vi "Server Client Loop.vi"(5 "TCPMessageAPI":refnum<class "TCPMessageAPI.lvclass">, 6 "Client Action Q":refnum<queue>, 7 "Fwd Queue":refnum<queue>, 8 "TCP Client":refnum<k5>, 9 "Remote Port":u16, 10 "Remote Address":string, 11 "Conn Handlers":refnum<queue>) -> ()   [LabVIEW 2020, in "Vecto.lvlib" / "TCPMessaging.lvclass"]
uses:
  TCPMessaging.lvclass
  TX Payload.ctl
  Client Action Data.ctl
  Client Action.ctl
  Client Info.ctl
  proto/TcpClientHello/Data.ctl
  TCPMessageService/TCPMessageAPI.lvclass
  TCPConnectionHandler/TCPConnectionHandler.lvclass
  Server Client State.ctl
  Connection State.ctl
  Vecto.lvlib
  proto/TcpClientHello/TcpClientHello.lvlib
panel:
  out "Client Hello":T1
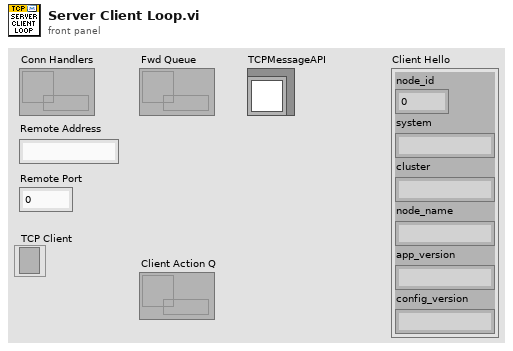
[diagram p1: front panel]
types:
  T1 = typedef "TcpClientHello.lvlib/Data.ctl" = cluster{"node_id":u32, "system":string, "cluster":string, "node_name":string, "app_version":string, "config_version":string}
  T2 = typedef "Vecto.lvlib/TCPMessaging.lvclass/Server Client State.ctl" = enum16{"Handshake", "Message", "Close"}
  T3 = enum16{"big-endian, network order", "native, host order", "little-endian"}
  T4 = typedef "Vecto.lvlib/TCPMessaging.lvclass/Client Action.ctl" = enum16{"Connect", "Ready", "Disconnect"}
  T5 = typedef "Vecto.lvlib/TCPMessaging.lvclass/Client Action Data.ctl" = cluster{"Client Action":T4, "Client Info":T6, "TCP":refnum<k5>, "TX Q":refnum<queue>}
  T6 = typedef "Vecto.lvlib/Client Info.ctl" = cluster{"TcpClientHello":T1, "Remote Address":string, "Remote Port":u16}
  T7 = typedef "Vecto.lvlib/Connection State.ctl" = enum16{"Connected", "Disconnected"}
  T8 = typedef "Vecto.lvlib/TX Payload.ctl" = cluster{"Target ID":u32, "Payload":string}
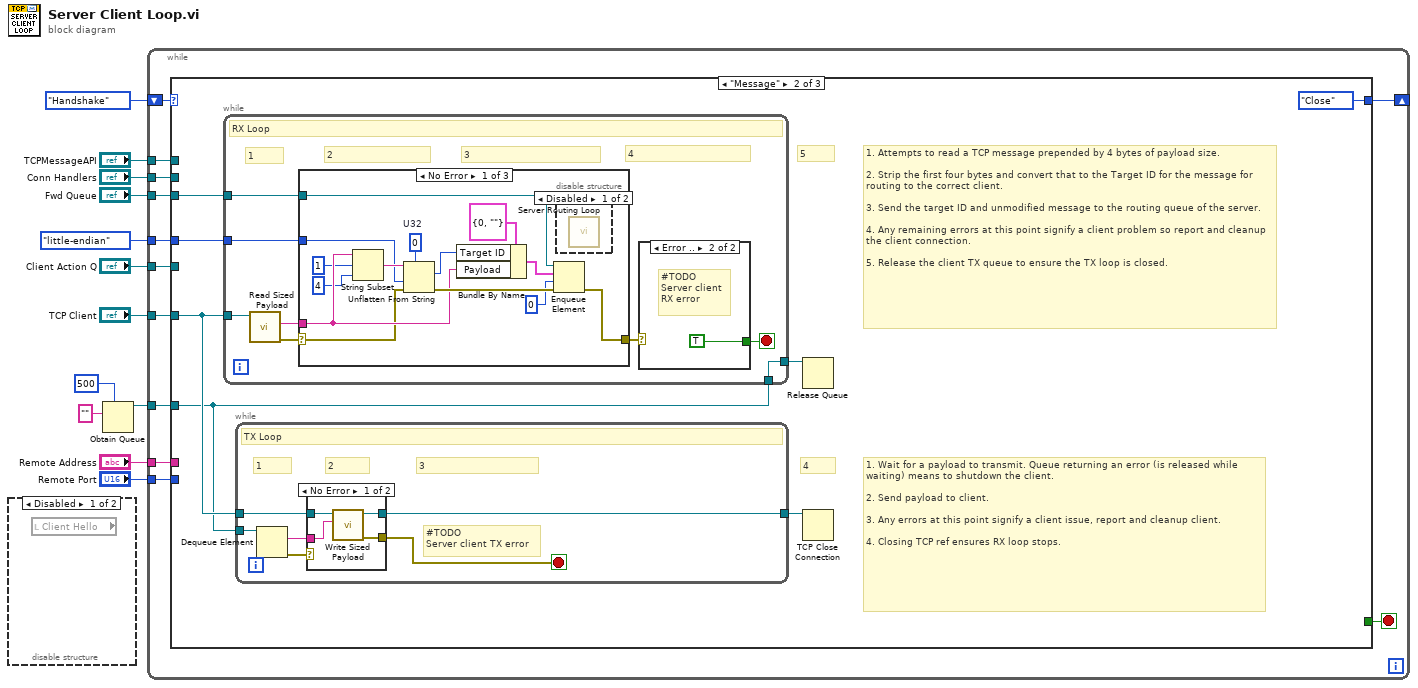
[diagram p0: block diagram]
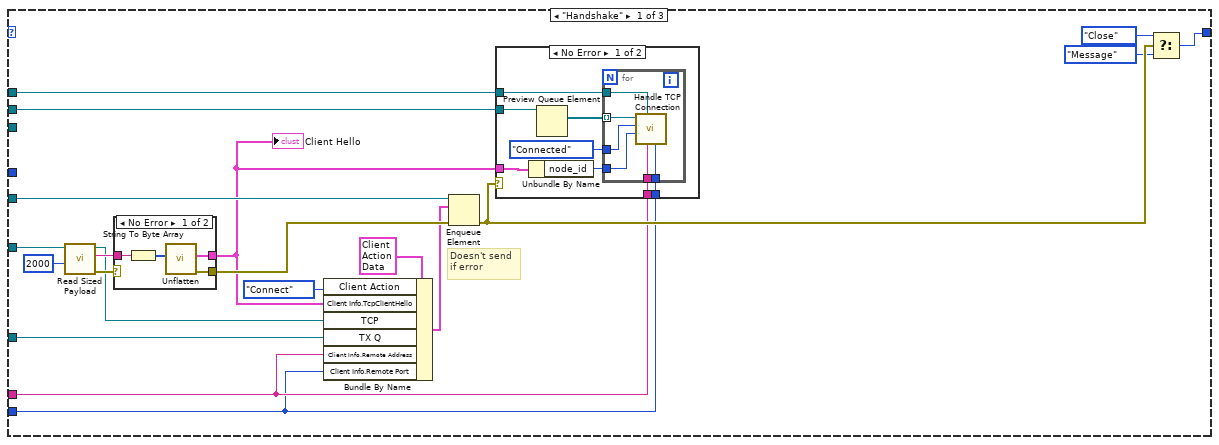
[diagram p3: hidden frame]
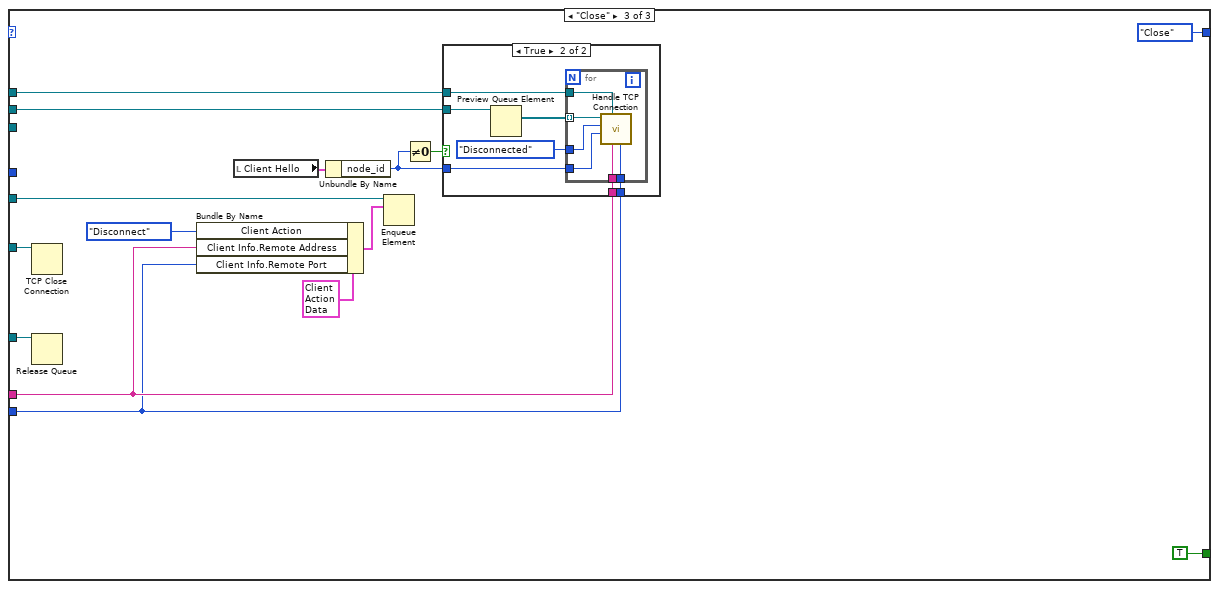
[diagram p11: hidden frame]
diagram:
  n1 = disable-structure shown="Disabled" {
    frame Disabled {
      n2 = local read "Client Hello"() -> ()  [unwired: 1 out]
    }
    frame Enabled {
    }
  }
  n3 = Obtain Queue(max queue size (-1, unlimited)=500, element data type="") -> (queue out=w4:refnum<queue>)  [unwired: 3 in, 2 out]
  n4 = while {
    tunnel: "Fwd Queue" -> [w24]
    tunnel: "TCP Client" -> [w23]
    tunnel: T3."little-endian" ("byte order (0:big-endian, network order)") -> [w22]
    shift-right: [w19] -> _
    shift-left: Server_Client_State."Handshake" ("Server Client State") -> [w20]
    tunnel: "Remote Address" -> [w18]
    tunnel: "Remote Port" -> [w17]
    tunnel: w4 -> [w16]
    tunnel: "Client Action Q" -> [w15]
    tunnel: "Conn Handlers" -> [w14]
    tunnel: "TCPMessageAPI" -> [w13]
    stop <- w21 stop-if-true
    n5 = case shown="\"Message\"" w20 {
      tunnel: w24 -> [_ w70 _]
      tunnel: w23 -> [w39 w69 w118]
      tunnel: w22 -> [_ w68 _]
      tunnel: [_ _ TRUE] -> w21
      tunnel: [w40 Server_Client_State."Close" ("Server Client State") Server_Client_State."Close" ("Server Client State")] -> w19
      tunnel: w18 -> [w26 _ w108]
      tunnel: w17 -> [w25 _ w107]
      tunnel: w16 -> [w30 w64 w119]
      tunnel: w15 -> [w35 _ w116]
      tunnel: w14 -> [w29 _ w113]
      tunnel: w13 -> [w28 _ w112]
      frame "Handshake" {
        # "Doesn't send if error"
        n6 = call "Read Sized Payload.vi"("timeout ms (100)"=2000, "TCP in"=w39) -> ("error out"=w37:errorcluster, "Payload"=w36:string, "TCP"=w32:refnum<k5>)  [unwired: 7 in]
        n7 = case shown="No Error" w37 {
          selector: w37 -> [_ w63]
          tunnel: w36 -> [w62 _]
          tunnel: [w60 _] -> w27
          tunnel: [w59 w63] -> w43
          frame No Error {
            n8 = String To Byte Array(string=w62) -> (unsigned byte array=w61:u8[])
            n9 = call "Unflatten.vi"("Buffer"=w61) -> ("error out"=w59:errorcluster, "Data"=w60:T1)  [unwired: 9 in]
          }
          frame Error {
          }
        }
        "Client Hello" <- w27
        n10 = Bundle By Name(cluster=T5 {"Client Action"=enum."Disconnect", "Client Info"={"TcpClientHello"={"node_id"=0, "system"="", "cluster"="", "node_name"="", "app_version"="", "config_version"=""}, "Remote Address"="", "Remote Port"=0}, "TCP"=refnum, "TX Q"=refnum} ("element"), "Client Action"=Client_Action."Connect", "Client Info.TcpClientHello"=w27, "TCP"=w32, "TX Q"=w30, "Client Info.Remote Address"=w26, "Client Info.Remote Port"=w25) -> (w31:T5)
        n11 = Enqueue Element(queue=w35, element=w31, error in (no error)=w43) -> (error out=w44:errorcluster)  [unwired: 1 in, 2 out]
        n12 = case shown="No Error" w44 {
          tunnel: w29 -> [w48 _]
          tunnel: w27 -> [w52 _]
          tunnel: w28 -> [w51 _]
          tunnel: w26 -> [w46 _]
          tunnel: w25 -> [w45 _]
          frame No Error {
            n13 = Unbundle By Name(w52) -> ("node_id"=w50:u32)
            n14 = Preview Queue Element(queue=w48) -> (element=w47:refnum<class "TCPConnectionHandler.lvclass">[])  [unwired: 2 in, 3 out]
            n15 = for {
              tunnel: w47 -> [w58] mode=indexing
              tunnel: w51 -> [w57]
              tunnel: w50 -> [w55]
              tunnel: Connection_State."Connected" ("Connection State") -> [w56]
              tunnel: w46 -> [w54]
              tunnel: w45 -> [w53]
              n16 = call-dynamic "Handle TCP Connection.vi"("Remote Port"=w53, "Remote Host"=w54, "TCPMessageAPI"=w57, "Node ID"=w55, "Connection State"=w56, "TCPConnectionHandler in"=w58) -> ()  [unwired: 4 in, 2 out]
            }
          }
          frame Error {
          }
        }
        n17 = Select(t=Server_Client_State."Close", s=w44, f=Server_Client_State."Message" ("Server Client State")) -> (s? t:f=w40:T2)
      }
      frame "Message" {
        # "4"
        # "5"
        # "1. Wait for a payload to transmit. Queue returning an error (is released while waiting) means to shutdown the client.\n\n2. Send payload to client.\n\n3. Any errors at this point signify a client issue, report and cleanup client.\n\n4. Closing TCP ref ensures RX loop stops."
        # "1. Attempts to read a TCP message prepended by 4 bytes of payload size.\n\n2. Strip the first four bytes and convert that to the Target ID for the message for routing to the correct client.\n\n3. Send the target ID and unmodified message to the routing queue of the server.\n\n4. Any remaining errors at this point signify a client problem so report and cleanup the client connection.\n\n5. Release the client TX queue to ensure the TX loop is closed."
        n18 = while {
          tunnel: w70 -> [w78]
          tunnel: w69 -> [w74]
          tunnel: w68 -> [w75]
          tunnel: w64 -> [w71]
          tunnel: [w71] -> w65
          stop <- w76 stop-if-true
          # "3"
          # "2"
          # "4"
          # "1"
          # "RX Loop"
          n19 = call "Read Sized Payload.vi"("TCP in"=w74) -> ("error out"=w73:errorcluster, "Payload"=w72:string)  [unwired: 8 in, 1 out]
          n20 = case shown="No Error" w73 {
            selector: w73 -> [w81 w93 _]
            tunnel: [w89 w93 _] -> w77
            tunnel: w78 -> [w91 _ _]
            tunnel: w75 -> [w83 _ _]
            tunnel: w72 -> [w82 _ _]
            frame No Error {
              w87 = u32 0  # U32
              n21 = String Subset(string=w82, offset (0)=1 ("length (rest)"), length (rest)=4 ("length (rest)")) -> (substring=w88:string)
              n22 = Unflatten From String(type=w87, binary string=w88, byte order (0:big-endian, network order)=w83, error in (no error)=w81) -> (value=w85:u32, error out=w92:errorcluster)  [unwired: 1 in, 1 out]
              n23 = Bundle By Name(cluster=T8 {"Target ID"=0, "Payload"=""} ("TX Payload"), "Target ID"=w85, "Payload"=w82) -> (w84:T8)
              n24 = Enqueue Element(queue=w91, element=w84, timeout in ms (-1)=0, error in (no error)=w92) -> (error out=w89:errorcluster)  [unwired: 2 out]
              n25 = disable-structure shown="Disabled" {
                frame Disabled {
                  n26 = call "Server Routing Loop.vi"() -> ()  [unwired: 11 in, 1 out]
                }
                frame Enabled {
                }
              }
            }
            frame Default {
            }
            frame Error {
              # "Timeout, don't propagate error to iterate again and wait another interval for data."
            }
          }
          n27 = case shown="Error .." w77 {
            tunnel: [_ TRUE] -> w76
            frame No Error {
            }
            frame Error {
              # "#TODO\nServer client RX error"
            }
          }
        }
        n28 = while {
          tunnel: w64 -> [w100]
          tunnel: w69 -> [w99]
          tunnel: [w96] -> w67
          stop <- w95 stop-if-true
          # "#TODO\nServer client TX error"
          # "3"
          # "2"
          # "1"
          # "TX Loop"
          n29 = Dequeue Element(queue=w100) -> (element=w98:string, error out=w97:errorcluster)  [unwired: 2 in, 2 out]
          n30 = case shown="No Error" w97 {
            selector: w97 -> [_ w105]
            tunnel: w99 -> [w103 w106]
            tunnel: w98 -> [w104 _]
            tunnel: [w101 w105] -> w95
            tunnel: [w102 w106] -> w96
            frame No Error {
              n31 = call "Write Sized Payload.vi"("Payload"=w104, "TCP in"=w103) -> ("error out"=w101:errorcluster, "TCP"=w102:refnum<k5>)  [unwired: 8 in]
            }
            frame Default {
            }
          }
        }
        n32 = Release Queue(queue=w65) -> ()  [unwired: 2 in, 3 out]
        n33 = TCP Close Connection(connection ID=w67) -> ()  [unwired: 2 in, 2 out]
      }
      frame "Close" {
        n34 = TCP Close Connection(connection ID=w118) -> ()  [unwired: 2 in, 2 out]
        n35 = Release Queue(queue=w119) -> ()  [unwired: 2 in, 3 out]
        n36 = Bundle By Name(cluster=T5 {"Client Action"=enum."Disconnect", "Client Info"={"TcpClientHello"={"node_id"=0, "system"="", "cluster"="", "node_name"="", "app_version"="", "config_version"=""}, "Remote Address"="", "Remote Port"=0}, "TCP"=refnum, "TX Q"=refnum} ("element"), "Client Action"=Client_Action."Disconnect", "Client Info.Remote Address"=w108, "Client Info.Remote Port"=w107) -> (w114:T5)
        n37 = local read "Client Hello"() -> (w111:T1)
        n38 = Unbundle By Name(w111) -> ("node_id"=w110:u32)
        n39 = Enqueue Element(queue=w116, element=w114) -> ()  [unwired: 2 in, 3 out]
        n40 = Not Equal To 0?(x=w110) -> (x != 0?=w109:bool)
        n41 = case shown="True" w109 {
          tunnel: w113 -> [_ w126]
          tunnel: w112 -> [_ w128]
          tunnel: w110 -> [_ w127]
          tunnel: w108 -> [_ w123]
          tunnel: w107 -> [_ w122]
          frame False {
          }
          frame True {
            n42 = Preview Queue Element(queue=w126) -> (element=w125:refnum<class "TCPConnectionHandler.lvclass">[])  [unwired: 2 in, 3 out]
            n43 = for {
              tunnel: w128 -> [w134]
              tunnel: w127 -> [w133]
              tunnel: w125 -> [w132] mode=indexing
              tunnel: Connection_State."Disconnected" ("Connection State") -> [w131]
              tunnel: w123 -> [w130]
              tunnel: w122 -> [w129]
              n44 = call-dynamic "Handle TCP Connection.vi"("Remote Port"=w129, "Remote Host"=w130, "TCPMessageAPI"=w134, "Node ID"=w133, "Connection State"=w131, "TCPConnectionHandler in"=w132) -> ()  [unwired: 4 in, 2 out]
            }
          }
        }
      }
    }
  }
